vi "http POST Message.vi"(1 "http Message Body":string) -> (0 "http POST Message":string)   [LabVIEW 2020, in "FT-IR.lvlib" / "TOOLweb Interface.lvlib" / "TOOLweb Interface Hilfs-VIs.lvlib"]
doc: "Erstellt den Header für einen http-Request nach der Methode \"POST\". \n\n\"http Message Body\": übernimmt einen String im Format einer XML-Text-Nachricht\n\"http POST Message\": liefert den sendefertigen http-Request-String"
uses:
  TOOLweb Interface Hilfs-VIs.lvlib
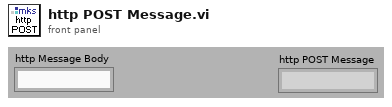
[diagram p1: front panel]
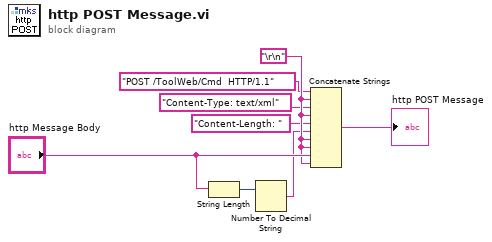
[diagram p0: block diagram]
diagram:
  w7 = "\r\n"
  n1 = String Length(string="http Message Body") -> (length=w5:i32)
  n2 = Number To Decimal String(number=w5) -> (decimal integer string=w6:string)  [unwired: 1 out]
  n3 = Concatenate Strings("POST /ToolWeb/Cmd  HTTP/1.1" ("Adresse"), w7, "Content-Type: text/xml" ("Adresse"), w7, "Content-Length: " ("Adresse"), w6, w7, w7, "http Message Body", w7) -> (→"http POST Message":string)
